vi "Cursor Set Unset Busy.vi"(8 "Set Busy? (F)":bool, 11 "Parent VI":refnum<vi>) -> ()   [LabVIEW 2016]
uses:
  VI Ref Global.vi
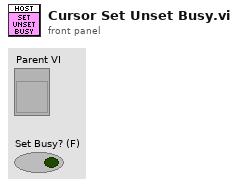
[diagram p1: front panel]
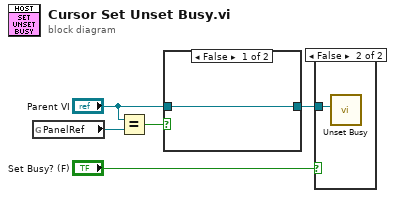
[diagram p0: block diagram]
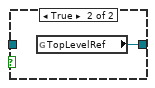
[diagram p2: hidden frame]
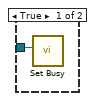
[diagram p3: hidden frame]
diagram:
  n1 = global read "VI Ref Global.vi" "PanelRef"() -> (w5:refnum<vi>)
  n2 = Equal?(x="Parent VI", y=w5) -> (x = y?=w4:bool)
  n3 = case shown="False" w4 {
    tunnel: [w6 w7] -> w2
    tunnel: "Parent VI" -> [w6 _]
    frame False {
    }
    frame True {
      n4 = global read "VI Ref Global.vi" "TopLevelRef"() -> (w7:refnum<vi>)
    }
  }
  n5 = case shown="False" "Set Busy? (F)" {
    tunnel: w2 -> [w8 w9]
    frame True {
      n6 = call <vilib>:"Set Busy.vi"("VI reference (current VI)"=w8) -> ()  [unwired: 9 in, 2 out]
    }
    frame False {
      n7 = call <vilib>:"Unset Busy.vi"("VI reference (current VI)"=w9) -> ()  [unwired: 10 in, 1 out]
    }
  }
